vi "Dispose DataBindings.vi"(8 "error in (no error)":errorcluster caption="错误输入（无错误）", 11 "OleDBClass 输入":refnum<class "OleDBClass.lvclass"> caption="DNL_LabVIEW Object in") -> (0 "error out":errorcluster caption="错误输出", 3 "OleDBClass 输出":refnum<class "OleDBClass.lvclass"> caption="DNL_LabVIEW Object out")   [LabVIEW 2012, in "OleDBClass.lvclass"]
uses:
  OleDBClass.lvclass
  OleDBClass.lvclass/OleDBClass.ctl
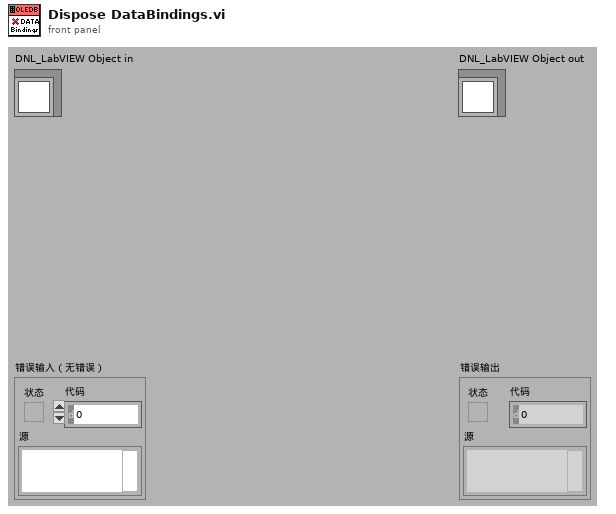
[diagram p1: front panel]
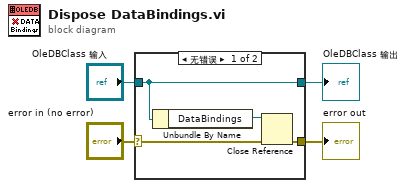
[diagram p0: block diagram]
diagram:
  n1 = case shown="无错误" "error in (no error)" {
    selector: "error in (no error)" -> [w7 w10]
    tunnel: [w6 w10] -> w3
    tunnel: [w8 w9] -> w1
    tunnel: "OleDBClass 输入" -> [w8 w9]
    frame No Error {
      n2 = Unbundle By Name(w8) -> ("DataBindings"=w5:refnum<k24>)
      n3 = Close Reference(reference=w5, error in (no error)=w7) -> (error out=w6:errorcluster)
    }
    frame Error {
    }
  }
  "error out" <- w3
  "OleDBClass 输出" <- w1
